vi "PCAN_SPECIAL_FUNKTION.vi"(8 "error in (no error)":errorcluster, 10 "codenumber":i16, 11 "distributorcode":u32) -> (0 "error out":errorcluster, 3 "failed":bool)   [LabVIEW 2016]
uses:
  PCAN_USB.DLL
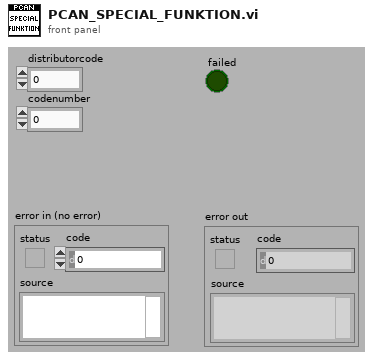
[diagram p1: front panel]
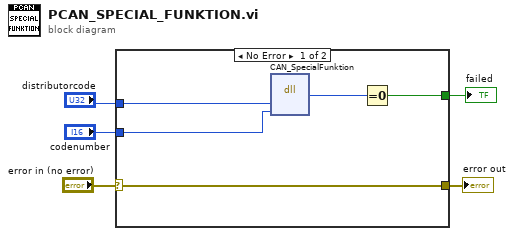
[diagram p0: block diagram]
diagram:
  n1 = case shown="No Error" "error in (no error)" {
    selector: "error in (no error)" -> [w10 w11]
    tunnel: [w10 w11] -> w3
    tunnel: "distributorcode" -> [w9 _]
    tunnel: "codenumber" -> [w8 _]
    tunnel: [w6 _] -> w1
    frame No Error {
      n2 = dll-call lib="D:/LabView/02_NI/PCAN_Driver/PCAN_USB.DLL" fn="CAN_SpecialFunktion"("distributorcode"=w9, "codenumber"=w8) -> (w7:i32)  [unwired: 5 in, 2 out]
      n3 = Equal To 0?(x=w7) -> (x = 0?=w6:bool)
    }
    frame Error {
    }
  }
  "error out" <- w3
  "failed" <- w1
